vi "niFpgaMemoryEmulationDramRetrieveDataRefIn.vi"(1 "Name":variant, 7 "data type":i32, 9 "ready for output":bool, 11 "error in (no error)":errorcluster, 12 "Node Link":cluster{"VIRef":refnum<vi>, "UID":i32}) -> (8 "data":i32, 10 "output valid":bool, 15 "error out":errorcluster)   [LabVIEW 2017]
uses:
  <vilib>/rvi/DataTransferAndStorage/Container/Common/niFpgaContainerMetaDataKey.ctl
  <instcachedir>/0/niFpgaMemoryEmulationDramRetrieveData_1E02CFB0A4FA4732866F8B6EB8630FB9.lvgen/niFpgaMemoryEmulationDramRetrieveData_1E02CFB0A4FA4732866F8B6EB8630FB9_000.vi
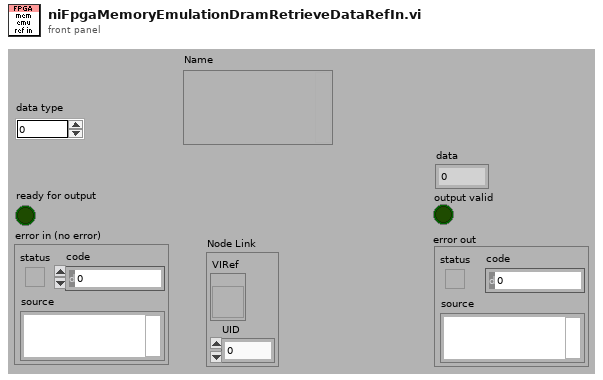
[diagram p1: front panel]
types:
  T1 = typedef "niFpgaContainerMetaDataKey.ctl" = enum16{"FPGA FIFO", "FPGA Memory", "FPGA Register", "FPGA Handshake"}
  T2 = typedef "niFpgaContainerState.ctl" = cluster{"displayName":string, "hardwareName":string, "dataType":T3, "elementTypeDescriptor":variant, "terminalTypeDescriptor":variant, "requestedNumberOfElements":u32, "memoryType":T4, "arbitrationForInterfaceA":T5, "numberOfElementsPerRead":u32, "arbitrationForInterfaceB":T5, "numberOfElementsPerWrite":u32, "VI_Defined":bool, "type":T6, "initializationParameters":T7, "disableOnOverflow/Underflow":bool, "interfaceConfiguration":T8, "controlLogic":T9, "actualNumberOfElements":u32, "dramSelection":string, "dramMaxOustandingRequests":i32, "dramIncludeByteEnables":bool, "dramGrantTime":u32, "fullEmulation":bool, "memoryInMultipleClockDomains":bool, "memoryLatency":T10}
  T3 = typedef "niFpgaDataTypeControl.ctl" = enum32{"Boolean", "I8", "I16", "I32", "I64", "U8", "U16", "U32", "U64", "FXP", "CustomControl", "SGL"}
  T4 = typedef "niFpgaContainerImplementationControl.ctl" = enum16{"Flip-Flops", "Look-Up Table", "Block Memory", "DRAM"}
  T5 = typedef "niFpgaContainerArbitrationOptionsControl.ctl" = enum16{"Always Arbitrate", "Arbitrate if Multiple Requestors Only", "Never Arbitrate"}
  T6 = typedef "niFpgaTransferTypeControl.ctl" = enum16{"Target-Scoped", "Host to Target - DMA", "Target to Host - DMA", "Peer to Peer Reader", "Peer to Peer Writer", "Bidirectional"}
  T7 = typedef "niFpgaContainerInitializationParameters.ctl" = cluster{"initialized":bool, "VI_Path":path, "initialData":variant}
  T8 = typedef "niFpgaMemoryInterfaceConfiguration.ctl" = enum16{"Read A-Write B", "Read A-Read B"}
  T9 = typedef "niFpgaFifoControlLogicControl.ctl" = enum16{"Slice Fabric", "Target Optimal", "Built-in"}
  T10 = typedef "niFpgaContainerMemoryLatencyControl.ctl" = u16
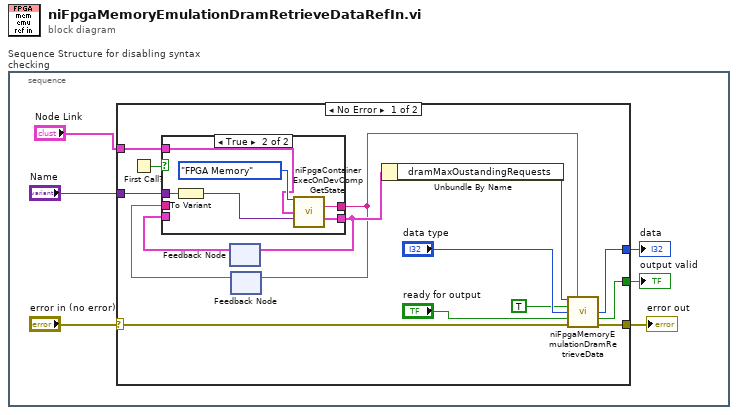
[diagram p0: block diagram]
diagram:
  n1 = stacked-sequence "Sequence Structure for disabling syntax checking" {
    frame #0 {
      n2 = case shown="No Error" "error in (no error)" {
        selector: "error in (no error)" -> [w12 w30]
        tunnel: [w21 w30] -> w2
        tunnel: "Name" -> [w18 _]
        tunnel: [w9 _] -> w5
        tunnel: [w8 _] -> w6
        tunnel: "Node Link" -> [w7 _]
        frame No Error {
          n3 = First Call?() -> (First Call?: T/F=w19:bool)
          n4 = feedback #1() -> (w15:T2)  [unwired: 1 out]
          n5 = feedback #2() -> (w13:string)  [unwired: 1 out]
          n6 = case shown="True" w19 {
            tunnel: w18 -> [_ w29]
            tunnel: [w23 w25] -> w16
            tunnel: w15 -> [w23 _]
            tunnel: [w22 w26] -> w14
            tunnel: w13 -> [w22 _]
            tunnel: w7 -> [_ w24]
            frame False {
            }
            frame True {
              n7 = To Variant(anything=w29) -> (Variant=w28:variant)
              n8 = call <vilib>:"niFpgaContainerExecOnDevCompGetState.vi"("containerMetaDataKey"=niFpgaContainerMetaDataKey."FPGA Memory", "Node Link"=w24, "name"=w28) -> ("Unique  Name"=w26:string, "containerState"=w25:T2)  [unwired: 3 in, 8 out]
            }
          }
          n9 = feedback-in #1(w16) -> ()
          n10 = feedback-in #2(w14) -> ()
          n11 = Unbundle By Name(w16) -> ("dramMaxOustandingRequests"=w11:i32)
          n12 = call-generic <vilib>:"niFpgaMemoryEmulationDramRetrieveData.vi"("fifo size"=w11, "name"=w14, "ref in wired"=TRUE, "data type"="data type", "ready for output"="ready for output", "error in (no error)"=w12) -> ("data"=w8:i32, "output valid"=w9:bool, "error out"=w21:errorcluster)  [unwired: 7 in]
        }
        frame Error {
        }
      }
      "error out" <- w2
      "output valid" <- w5
      "data" <- w6
    }
  }
